vi "Config Data Get Key Value.vi"(0 "config data":T1 caption="Konfigurationsdaten", 1 "section":string caption="Abschnitt", 5 "key":string caption="Schlüssel", 11 "error in (no error)":errorcluster caption="Fehler (Eingang, kein Fehler)") -> (3 "section exists?":bool caption="Abschnitt vorhanden?", 4 "config data out":T1 caption="Konfigurationsdaten (Ausgang)", 6 "key exists?":bool caption="Schlüssel vorhanden?", 10 "key value":string caption="Schlüsselwert", 13 "key index":i32 caption="Schlüsselindex", 15 "error out":errorcluster caption="Fehler (Ausgang)")   [LabVIEW 2009]
doc: "Ermittelt, ob ein Schlüssel in einem angegebenen Abschnitt eines Konfigurationsdatenobjekts existiert."
uses:
  <vilib>/Utility/config.llb/Config Data RefNum.ctl
  Config Data Registry Functions.ctl
  <vilib>/Utility/config.llb/NI_LVConfig.lvlib
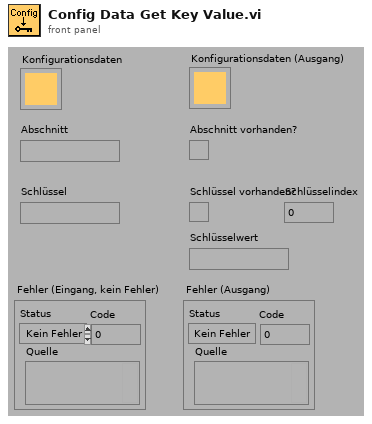
[diagram p1: front panel]
types:
  T1 = typedef "NI_LVConfig.lvlib/Config Data RefNum.ctl" = refnum<k1>
  T2 = typedef "Config Data Registry Functions.ctl" = enum16{"reset", "register", "get data", "get section", "set data", "unregister", "test", "get objects"}
  T3 = typedef "Config Data Section.ctl" = cluster{"keys":string[], "values":string[]}
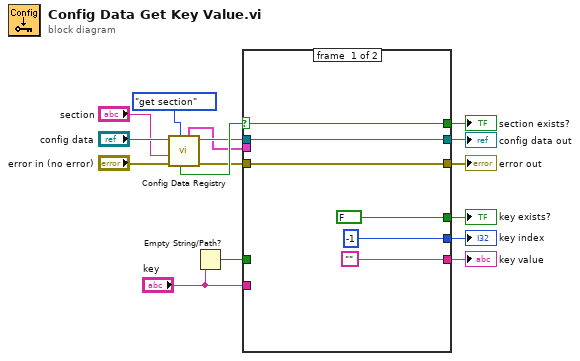
[diagram p0: block diagram]
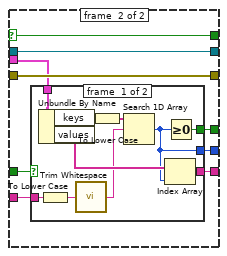
[diagram p2: hidden frame]
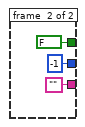
[diagram p3: hidden frame]
diagram:
  n1 = call "Config Data Registry.vi"("function (get data)"=Config_Data_Registry_Functions."get section", "error in (no error)"="error in (no error)", "section"="section", "config data"="config data") -> ("error out"=w5:errorcluster, "config data out"=w7:T1, "section"=w6:T3, "valid section?"=w9:bool)  [unwired: 1 in, 3 out]
  n2 = Empty String/Path?(string/path="key") -> (empty?=w1:bool)
  n3 = case shown="True" w9 {
    selector: w9 -> [w22 w31]
    tunnel: [w22 w31] -> w16
    tunnel: [FALSE w30] -> w15
    tunnel: w7 -> [w20 w29]
    tunnel: w5 -> [w19 w28]
    tunnel: [w19 w28] -> w13
    tunnel: [w20 w29] -> w14
    tunnel: w6 -> [_ w25]
    tunnel: ["" w27] -> w12
    tunnel: [-1 ("index of element") w26] -> w11
    tunnel: "key" -> [_ w23]
    tunnel: w1 -> [_ w24]
    frame #0 {
    }
    frame #1 {
      n4 = case shown="False" w24 {
        tunnel: [w40 FALSE] -> w30
        tunnel: [w38 ""] -> w27
        tunnel: [w37 -1 ("index of element")] -> w26
        tunnel: w25 -> [w36 _]
        tunnel: w23 -> [w35 _]
        frame #0 {
          n5 = Unbundle By Name(w36) -> ("keys"=w41:string[], "values"=w39:string[])
          n6 = To Lower Case(string=w35) -> (all lower case string=w33:string)
          n7 = call "Trim Whitespace.vi"("string"=w33) -> ("trimmed string"=w32:string)  [unwired: 1 in]
          n8 = To Lower Case(string=w41) -> (all lower case string=w34:string[])
          n9 = Search 1D Array(1D array=w34, element=w32) -> (index of element=w37:i32)  [unwired: 1 in]
          n10 = Index Array(array=w39, index=w37) -> (element=w38:string)
          n11 = Greater Or Equal To 0?(x=w37) -> (x >= 0?=w40:bool)
        }
        frame #1 {
        }
      }
    }
  }
  "config data out" <- w14
  "error out" <- w13
  "section exists?" <- w16
  "key exists?" <- w15
  "key value" <- w12
  "key index" <- w11
